vi "get_motion_by_name.vi"(8 "error in (no error)":errorcluster caption="错误输入（无错误）", 10 "name":string, 11 "MotorSystem in":refnum<class "MotorSystem.lvclass">) -> (0 "error out":errorcluster caption="错误输出", 2 "motion cluster":T1, 3 "MotorSystem out":refnum<class "MotorSystem.lvclass">)   [LabVIEW 2016, in "MotionControl_UFO_3DOF.lvlib" / "MotorSystem.lvclass"]
uses:
  <userlib>/MotionControl_UFO_3DOF/MotorSystem/MotorSystem.lvclass
  <userlib>/MotionControl_UFO_3DOF/MotorSystem/MotionCluster.ctl
  <userlib>/MotionControl_UFO_3DOF/OneMotion/OneMotion.lvclass
  <userlib>/MotionControl_UFO_3DOF/MotorSystem/MotorSystem.lvclass/MotorSystem.ctl
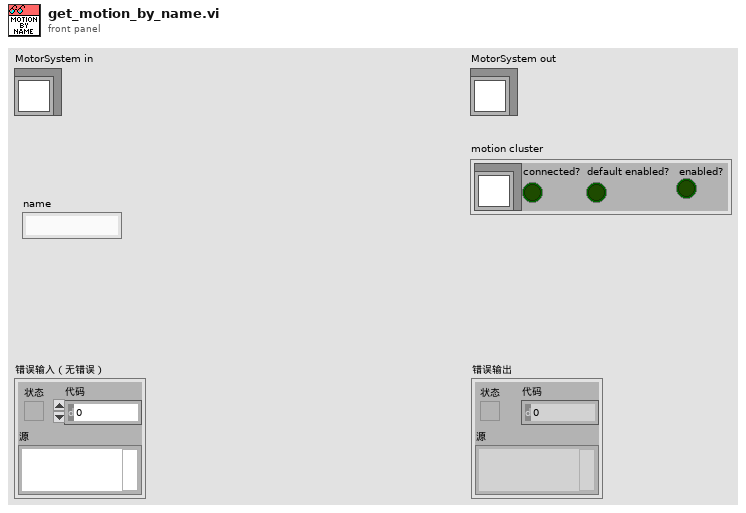
[diagram p1: front panel]
types:
  T1 = typedef "MotionControl_UFO_3DOF.lvlib/MotorSystem.lvclass/MotionCluster.ctl" = cluster{"OneMotion.lvclass":refnum<class "OneMotion.lvclass">, "connected?":bool, "default enabled?":bool, "enabled?":bool}
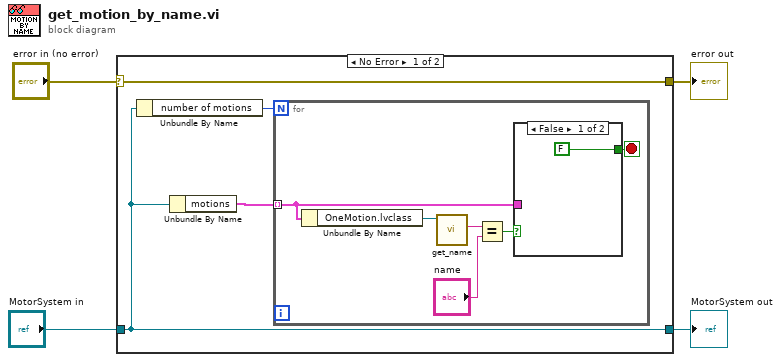
[diagram p0: block diagram]
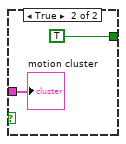
[diagram p2: hidden frame]
diagram:
  n1 = case shown="No Error" "error in (no error)" {
    selector: "error in (no error)" -> [w8 w18]
    tunnel: [w8 w18] -> w3
    tunnel: [w7 w19] -> w1
    tunnel: "MotorSystem in" -> [w7 w19]
    frame No Error {
      n2 = Unbundle By Name(w7) -> ("number of motions"=w6:i32)
      n3 = Unbundle By Name(w7) -> ("motions"=w5:T1[])
      n4 = for {
        N: w6 -> [_]
        tunnel: w5 -> [w10] mode=indexing
        stop <- w9 stop-if-true
        n5 = Unbundle By Name(w10) -> ("OneMotion.lvclass"=w14:refnum<class "OneMotion.lvclass">)
        n6 = call-dynamic "get_name.vi"("OneMotion输入"=w14) -> ("name"=w13:string)  [unwired: 8 in, 2 out]
        n7 = Equal?(x=w13, y="name") -> (x = y?=w11:bool)
        n8 = case shown="False" w11 {
          tunnel: w10 -> [_ w17]
          tunnel: [FALSE TRUE] -> w9
          frame False {
          }
          frame True {
            "motion cluster" <- w17
          }
        }
      }
    }
    frame Error {
    }
  }
  "error out" <- w3
  "MotorSystem out" <- w1
